vi "Programa_robot_final_2_condicionMala.vi"() -> ()   [LabVIEW 2019]
uses:
  <vilib>/Instr/_visa.llb/VISA Configure Serial Port (Instr).vi
  Global_STOP.vi
  <vilib>/regexp/Match Regular Expression.xnode
panel:
  out "error out":errorcluster
  in  "STOP TEST 2":bool
  out "Datos_QR 2":string
  out "NUMERO ASICS TESTEADOS":i32
  out "Existe foto anterior?":bool
  out ".not. x?":bool
  in  "Config File":path=path "C:/Trabajo/Test Asic Javi_2021/Origen Socket SERVO_PCB_BUENO_v5 (muchos asics)/CONFIG/configuracion_robot_CTAV2022A.test"
  in  "SELECCION DE TEST":string(combo)
  in  "?":bool
  out "Boolean":bool
  in  "Cerrar socket":bool
  in  "Abrir socket":bool
  out "Error_QR":bool
  in  "Interruptor Error":bool
  in  "stop socket 2":bool
  out "Bytes at port 3":u32=1
  in  "IN y":string(combo)="08"
  in  "IN x":string(combo)="06"
  in  "NOK y":string(combo)="00"
  in  "NOK x":string(combo)="00"
  in  "OK y":string(combo)="00"
  in  "OK x":string(combo)="00"
  in  "Operator's name":string(combo)="Juan Rodríguez"
  in  "?":bool
  in  "Fichero de registro":path=path "C:/Trabajo/Pruebas/Pruebas.txt"
  in  "Path Out Report":path=path "C:/Trabajo"
  out "Datos_QR":string
  in  "stop socket":bool
  out "Bytes at port 1":u32
  out "Iteraciones":i32
  out "Lectura buffer":string="1"
  in  "Delay (ms)":dbl=1.0 min=1.0 max=9.0 step=1.0
  out "Bytes at port 2":u32=1
  out "message":string=" INSTRUCTIONS:\r\rNormal Use:  When using subVIs that incorporate the error in/error out (or error I/O) structure, place this handler where you want to inform the user of an error, typically at the end of the I/O data path, as the last action of the program.  If the error in error? is ERROR, the handler creates a message describing the error and its source.  If the type of dialog = 1 (default), the message is displayed to the user, who can only acknowedge it.  If the type = 2, the user can acknowledge the message or abort execution; aborting a program with active I/O is not recommended.  If the type = 0, no message is displayed; this is used to process the error programmatically, and the error out cluster elements are wired to individual terminals for that reason.  \r\rOther Use:\n\r\nlocal testing.  To test the error code of a subVI or function that does not have the error I/O structure, you can wire its error code and a source string to the local error code and error source inputs.  If error in error? indicates no error and error code is not equal to 0, the local code and source are substituted for the error in values, and error? is set TRUE (ERROR)."
  in  "Interruptor":bool=TRUE
  in  "stop":bool
  # "Funcionamiento: en la primera iteración, el efector se desplaza desde el origen hasta la celda\nintroducida, hace una pausa, va a la posición del socket (0,0), hace otra pausa, va a la celda\nde salida y vuelve al origen. En las iteraciones siguientes hará lo mismo pero recorriendo las\nceldas de la bandeja sucesivamente. Que el desplazamiento se produzca hacia una celda de\nla bandeja OK o de la bandeja NOK depende de la salidad del programa de test de Asics."
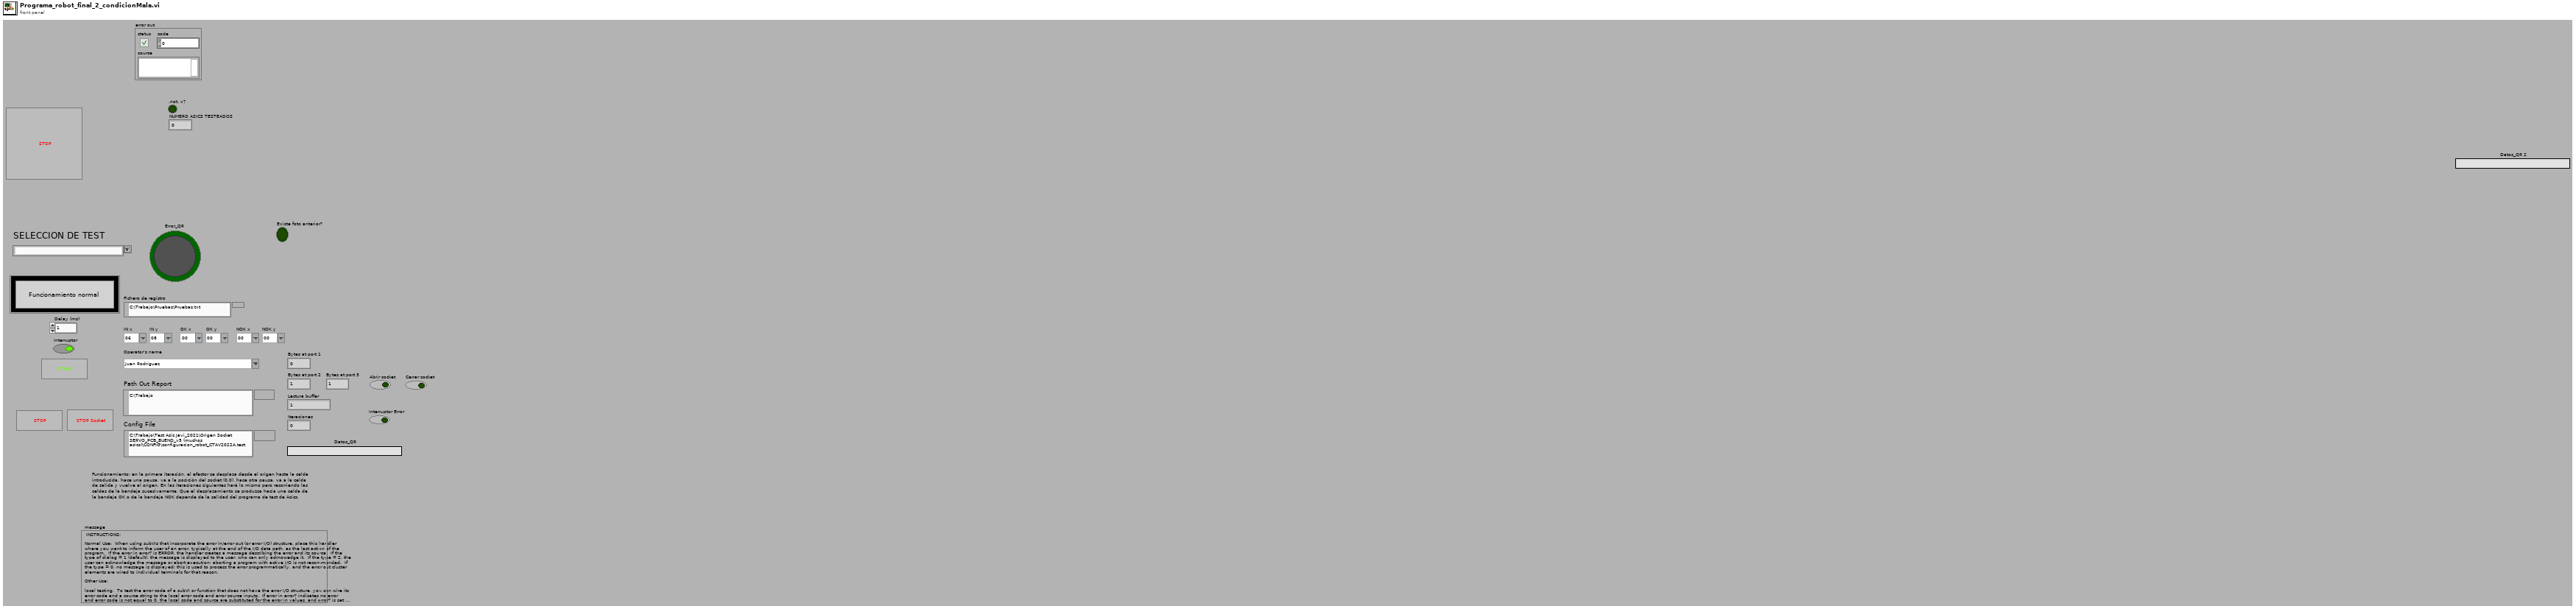
[diagram p1: front panel]
types:
  T1 = enum16{"open", "replace", "create", "open or create", "replace or create", "replace or create with confirmation"}
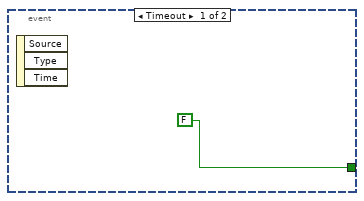
[diagram p2: hidden frame]
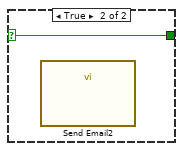
[diagram p3: hidden frame]
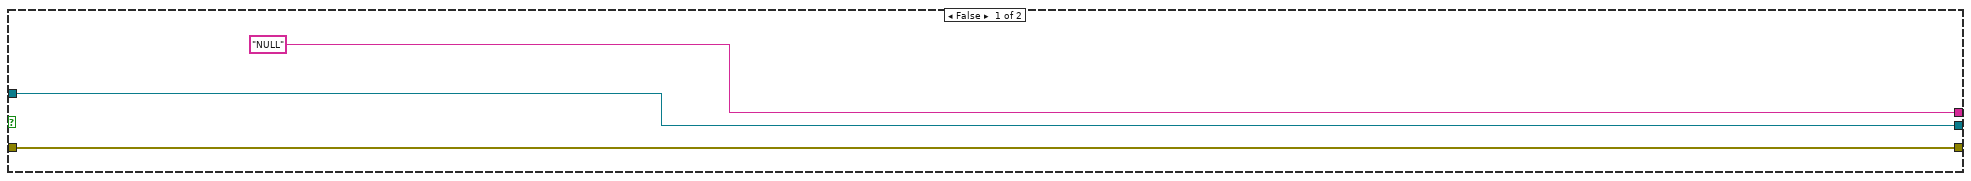
[diagram p4: hidden frame]
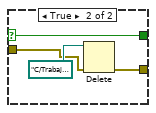
[diagram p7: hidden frame]
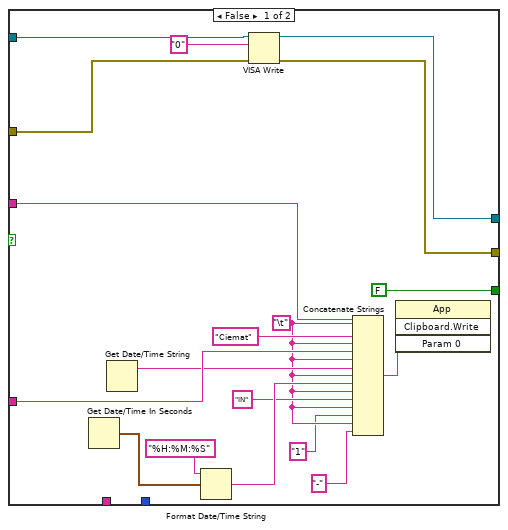
[diagram p9: hidden frame]
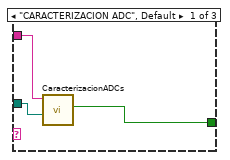
[diagram p10: hidden frame]
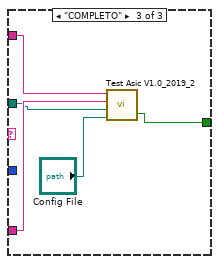
[diagram p11: hidden frame]
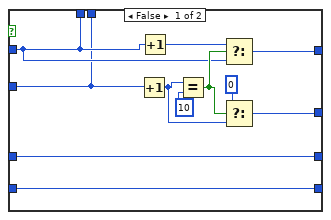
[diagram p13: hidden frame]
diagram:
  # "En el bucle de \"Enviar\" hay que cambiar a modo Latch y quitar la\nnegación para volver al funcionamiento original en el que se avanza\nuna iteración al presionar el botón."
  n1 = flat-sequence {
    tunnel: [w43] -> w5
    tunnel: ["Fichero de registro"] -> w4
    tunnel: ["SELECCION DE TEST"] -> w3
    tunnel: ["NOK y"] -> w20
    tunnel: ["NOK x"] -> w19
    tunnel: ["OK y"] -> w18
    tunnel: ["OK x"] -> w17
    tunnel: ["IN y"] -> w16
    tunnel: ["IN x"] -> w15
    tunnel: [w46] -> w14
    tunnel: [w47] -> w13
    tunnel: ["IN y"] -> w12
    tunnel: ["IN x"] -> w11
    tunnel: w4 -> [w45]
    frame #0 {
      n2 = while {
        stop <- w37 stop-if-true
        n3 = global read "Global_STOP.vi" "stop"() -> (w39:bool)
        n4 = Not(x="?") -> (.not. x?=w40:bool)
        "Boolean" <- w40
        n5 = property on="Boolean" class="Bool (strict)"("Blinking"=w40) -> ()  [unwired: 2 in, 2 out]
        n6 = Or(x="?", y=w39) -> (x .or. y?=w37:bool)
      }
    }
    frame #1 {
      n7 = Not(x="?") -> (.not. x?=w43:bool)
      ".not. x?" <- w43
    }
    frame #2 {
      n8 = Open/Create/Replace File(file path (use dialog)=w45, operation (0:open)=T1."open", access (0:read/write)=enum16{"read/write", "read-only", "write-only"}."write-only") -> (refnum out=w58:refnum<file>, error out=w60:errorcluster)  [unwired: 3 in, 1 out]
      n9 = Set File Position(refnum=w58, from (0:start)=enum16{"start", "end", "current"}."end", error in=w60) -> (refnum out=w59:refnum<file>, error out=w61:errorcluster)  [unwired: 1 in]
      n10 = Write to Text File(file (use dialog)=w59, text="\r\n", error in=w61) -> (refnum out=w47:refnum<file>, error out=w46:errorcluster)  [unwired: 1 in, 1 out]
    }
  }
  n11 = Decimal String To Number(string=w12) -> (number=w10:i32)  [unwired: 2 in, 1 out]
  n12 = Decimal String To Number(string=w11) -> (number=w7:i32)  [unwired: 2 in, 1 out]
  n13 = Multiply(x=10, y=w10) -> (x*y=w8:i32)
  n14 = Decimal String To Number(string=w18) -> (number=w22:i32)  [unwired: 2 in, 1 out]
  n15 = Decimal String To Number(string=w17) -> (number=w21:i32)  [unwired: 2 in, 1 out]
  n16 = Decimal String To Number(string=w20) -> (number=w24:i32)  [unwired: 2 in, 1 out]
  n17 = Decimal String To Number(string=w19) -> (number=w23:i32)  [unwired: 2 in, 1 out]
  n18 = call-poly "VISA Configure Serial Port"("VISA resource name"=refnum<visa-resource-name> "COM4", "baud rate (9600)"=u32 9600, "data bits (8)"=u16 8) -> ("VISA resource name out"=w28:refnum<visa-resource-name>, "error out"=w31:errorcluster)  [unwired: 11 in]
  n19 = Add(x=w8, y=w7) -> (x+y=w6:i32)
  n20 = while {
    shift-right: [w70] -> w29
    shift-left: w31 -> [w112]
    tunnel: w28 -> [w110]
    tunnel: [w73] -> w30
    tunnel: w13 -> [w103]
    tunnel: [w102] -> w27
    tunnel: w14 -> [w101]
    tunnel: [w100] -> w26
    tunnel: w15 -> [w98]
    tunnel: w16 -> [w97]
    tunnel: w17 -> [w96]
    tunnel: w18 -> [w95]
    tunnel: w19 -> [w94]
    tunnel: w20 -> [w93]
    shift-right: [w86] -> _
    shift-left: w24 -> [w92]
    shift-right: [w88] -> _
    shift-left: w23 -> [w91]
    shift-right: [w85] -> _
    shift-left: w22 -> [w90]
    shift-right: [w87] -> _
    shift-left: w21 -> [w89]
    tunnel: w6 -> [w84]
    tunnel: w5 -> [w76]
    tunnel: w3 -> [w75]
    tunnel: [w68] -> w1
    i -> [w74]
    stop <- w68 stop-if-true
    # "Poner Sonda en glbal stop"
    n21 = flat-sequence {
      tunnel: w112 -> [w155]
      tunnel: w110 -> [w144]
      tunnel: [w146] -> w109
      tunnel: [w145] -> w108
      tunnel: w98 -> [w125]
      tunnel: w97 -> [w124]
      tunnel: w96 -> [w123]
      tunnel: w95 -> [w122]
      tunnel: w94 -> [w121]
      tunnel: w93 -> [w120]
      tunnel: w109 -> [w898]
      tunnel: w108 -> [w897]
      tunnel: [w896] -> w83
      tunnel: [w895] -> w81
      tunnel: [w894] -> _
      tunnel: w83 -> [w916]
      tunnel: [w914] -> w82
      tunnel: w81 -> [w915]
      tunnel: [w913] -> w80
      tunnel: w82 -> [w936]
      tunnel: w80 -> [w935]
      tunnel: w74 -> [w937]
      tunnel: [w933] -> w79
      tunnel: [w932] -> w78
      tunnel: [w931] -> w77
      tunnel: w74 -> [w1058]
      tunnel: [w1060] -> w106
      tunnel: [w1059] -> w105
      tunnel: [w1056] -> w99
      tunnel: w79 -> [w1055]
      tunnel: w78 -> [w1054]
      tunnel: w77 -> [w1053]
      tunnel: w76 -> [w1050]
      tunnel: w75 -> [w1048]
      tunnel: w74 -> [w1047]
      tunnel: [w1120] -> w104
      tunnel: [w1122] -> w107
      tunnel: w106 -> [w1121]
      tunnel: w105 -> [w1119]
      tunnel: w103 -> [w1126]
      tunnel: [w1125] -> w102
      tunnel: w101 -> [w1124]
      tunnel: [w1123] -> w100
      tunnel: w74 -> [w1116]
      tunnel: w99 -> [w1115]
      tunnel: w92 -> [w1111]
      tunnel: w91 -> [w1114]
      tunnel: w90 -> [w1113]
      tunnel: w89 -> [w1112]
      tunnel: [w1110] -> w86
      tunnel: [w1109] -> w88
      tunnel: [w1108] -> w85
      tunnel: [w1107] -> w87
      tunnel: w84 -> [w1106]
      tunnel: w74 -> [w1105]
      tunnel: [w1104] -> _
      frame #0 {
        n22 = for {
          N: 2 -> [_]
          shift-right: [w773] -> _
          shift-left: w125 -> [w778]
          shift-right: [w776] -> w141
          shift-left: w144 -> [w777]
          shift-right: [w774] -> w140
          shift-left: w155 -> [w775]
          stop <- w771 stop-if-true
          n23 = xnode "Match Regular Expression"("input string"=w778, "regular expression"="-?\\d") -> ("whole match"=w772:string, "after match"=w773:string)  [unwired: 4 in, 3 out]
          n24 = global read "Global_STOP.vi" "stop"() -> (w771:bool)
          n25 = VISA Write(VISA resource name=w777, write buffer=w772, error in (no error)=w775) -> (VISA resource name out=w776:refnum<visa-resource-name>, error out=w774:errorcluster)  [unwired: 1 out]
        }
        n26 = for {
          N: 2 -> [_]
          shift-right: [w650] -> _
          shift-left: w124 -> [w655]
          shift-right: [w653] -> w135
          shift-left: w141 -> [w654]
          shift-right: [w651] -> w134
          shift-left: w140 -> [w652]
          stop <- w648 stop-if-true
          n27 = xnode "Match Regular Expression"("input string"=w655, "regular expression"="-?\\d") -> ("whole match"=w649:string, "after match"=w650:string)  [unwired: 4 in, 3 out]
          n28 = global read "Global_STOP.vi" "stop"() -> (w648:bool)
          n29 = VISA Write(VISA resource name=w654, write buffer=w649, error in (no error)=w652) -> (VISA resource name out=w653:refnum<visa-resource-name>, error out=w651:errorcluster)  [unwired: 1 out]
        }
        n30 = for {
          N: 2 -> [_]
          shift-right: [w527] -> _
          shift-left: w123 -> [w532]
          shift-right: [w530] -> w137
          shift-left: w135 -> [w531]
          shift-right: [w528] -> w136
          shift-left: w134 -> [w529]
          stop <- w525 stop-if-true
          n31 = xnode "Match Regular Expression"("input string"=w532, "regular expression"="-?\\d") -> ("whole match"=w526:string, "after match"=w527:string)  [unwired: 4 in, 3 out]
          n32 = global read "Global_STOP.vi" "stop"() -> (w525:bool)
          n33 = VISA Write(VISA resource name=w531, write buffer=w526, error in (no error)=w529) -> (VISA resource name out=w530:refnum<visa-resource-name>, error out=w528:errorcluster)  [unwired: 1 out]
        }
        n34 = for {
          N: 2 -> [_]
          shift-right: [w404] -> _
          shift-left: w122 -> [w409]
          shift-right: [w407] -> w129
          shift-left: w137 -> [w408]
          shift-right: [w405] -> w128
          shift-left: w136 -> [w406]
          stop <- w402 stop-if-true
          n35 = xnode "Match Regular Expression"("input string"=w409, "regular expression"="-?\\d") -> ("whole match"=w403:string, "after match"=w404:string)  [unwired: 4 in, 3 out]
          n36 = global read "Global_STOP.vi" "stop"() -> (w402:bool)
          n37 = VISA Write(VISA resource name=w408, write buffer=w403, error in (no error)=w406) -> (VISA resource name out=w407:refnum<visa-resource-name>, error out=w405:errorcluster)  [unwired: 1 out]
        }
        n38 = for {
          N: 2 -> [_]
          shift-right: [w281] -> _
          shift-left: w121 -> [w286]
          shift-right: [w284] -> w131
          shift-left: w129 -> [w285]
          shift-right: [w282] -> w130
          shift-left: w128 -> [w283]
          stop <- w279 stop-if-true
          n39 = xnode "Match Regular Expression"("input string"=w286, "regular expression"="-?\\d") -> ("whole match"=w280:string, "after match"=w281:string)  [unwired: 4 in, 3 out]
          n40 = global read "Global_STOP.vi" "stop"() -> (w279:bool)
          n41 = VISA Write(VISA resource name=w285, write buffer=w280, error in (no error)=w283) -> (VISA resource name out=w284:refnum<visa-resource-name>, error out=w282:errorcluster)  [unwired: 1 out]
        }
        n42 = for {
          N: 2 -> [_]
          shift-right: [w158] -> _
          shift-left: w120 -> [w163]
          shift-right: [w161] -> w127
          shift-left: w131 -> [w162]
          shift-right: [w159] -> w126
          shift-left: w130 -> [w160]
          stop <- w156 stop-if-true
          n43 = xnode "Match Regular Expression"("input string"=w163, "regular expression"="-?\\d") -> ("whole match"=w157:string, "after match"=w158:string)  [unwired: 4 in, 3 out]
          n44 = global read "Global_STOP.vi" "stop"() -> (w156:bool)
          n45 = VISA Write(VISA resource name=w162, write buffer=w157, error in (no error)=w160) -> (VISA resource name out=w161:refnum<visa-resource-name>, error out=w159:errorcluster)  [unwired: 1 out]
        }
        n46 = Number To Decimal String(number="Delay (ms)") -> (decimal integer string=w149:string)  [unwired: 1 in]
        n47 = VISA Write(VISA resource name=w127, write buffer=w149, error in (no error)=w126) -> (VISA resource name out=w151:refnum<visa-resource-name>, error out=w150:errorcluster)  [unwired: 1 out]
        n48 = Select(t="1" ("write buffer"), s="Interruptor", f="0" ("write buffer")) -> (s? t:f=w147:string)
        n49 = VISA Write(VISA resource name=w151, write buffer=w147, error in (no error)=w150) -> (VISA resource name out=w146:refnum<visa-resource-name>, error out=w145:errorcluster)  [unwired: 1 out]
      }
      frame #1 {
        n50 = while {
          shift-right: [w906] -> w895
          shift-left: w897 -> [w911]
          tunnel: ["stop socket"] -> _
          shift-right: [w907] -> w896
          shift-left: w898 -> [w912]
          tunnel: ["stop socket"] -> w894
          stop <- w899 stop-if-true
          n51 = property class="Instr"(reference=w912, error in=w911) -> (reference out=w910:refnum<visa-resource-name>, error out=w909:errorcluster, "Bytes at Port"=w908:u32)
          "Bytes at port 1" <- w908
          n52 = VISA Read(VISA resource name=w910, byte count=w908, error in (no error)=w909) -> (VISA resource name out=w907:refnum<visa-resource-name>, read buffer=w905:string, error out=w906:errorcluster)  [unwired: 1 out]
          n53 = Equal?(x="2", y=w905) -> (x = y?=w903:bool)
          n54 = global read "Global_STOP.vi" "stop"() -> (w900:bool)
          n55 = Or(x=w903, y="stop socket") -> (x .or. y?=w901:bool)
          n56 = Compound Arithmetic op=OR(w901, w900) -> (w899:bool)
        }
      }
      frame #2 {
        n57 = while {
          shift-right: [w924] -> w913
          shift-left: w915 -> [w929]
          tunnel: ["stop socket 2"] -> _
          shift-right: [w925] -> w914
          shift-left: w916 -> [w930]
          tunnel: ["stop socket 2"] -> _
          stop <- w917 stop-if-true
          n58 = property class="Instr"(reference=w930, error in=w929) -> (reference out=w928:refnum<visa-resource-name>, error out=w927:errorcluster, "Bytes at Port"=w926:u32)
          "Bytes at port 3" <- w926
          n59 = VISA Read(VISA resource name=w928, byte count=w926, error in (no error)=w927) -> (VISA resource name out=w925:refnum<visa-resource-name>, read buffer=w923:string, error out=w924:errorcluster)  [unwired: 1 out]
          n60 = Equal?(x="3", y=w923) -> (x = y?=w921:bool)
          n61 = global read "Global_STOP.vi" "stop"() -> (w918:bool)
          n62 = Or(x=w921, y="stop socket 2") -> (x .or. y?=w919:bool)
          n63 = Compound Arithmetic op=OR(w919, w918) -> (w917:bool)
        }
      }
      frame #3 {
        # "Captura y lectura de QR"
        n64 = Greater?(x=w937, y=-1) -> (0:w934:bool)
        n65 = case shown="True" w934 {
          tunnel: [w941 w944] -> w931
          tunnel: w936 -> [w941 w945]
          tunnel: [w940 w943] -> w933
          tunnel: w935 -> [w940 w942]
          tunnel: ["NULL" ("Datos_QR") w946] -> w932
          frame False {
          }
          frame True {
            n66 = while {
              tunnel: [w965] -> w946
              tunnel: w945 -> [w964]
              tunnel: [w960] -> w944
              tunnel: [w959] -> w943
              tunnel: w942 -> [w955]
              stop <- w949 stop-if-true
              n67 = flat-sequence {
                tunnel: w955 -> [w967]
                tunnel: [w968] -> w954
                tunnel: [w981] -> w965
                tunnel: [w979] -> w956
                tunnel: [w978] -> w953
                tunnel: w954 -> [w978]
                frame #0 {
                  n68 = call <vilib>:"Check if File or Folder Exists.vi"("error in (no error)"=w967, "path"=path "C:/Trabajo/Test Asic Javi_2021/Origen Socket SERVO_PCB_BUENO_v5 (muchos asics)/capturaQR.jpg" ("path (use dialog)")) -> ("error out"=w966:errorcluster, "file or folder exists?"=w970:bool, "dup path"=w969:path)  [unwired: 7 in]
                  "Existe foto anterior?" <- w970
                  n69 = case shown="True" w970 {
                    tunnel: w969 -> [w973 w977]
                    tunnel: [w973 w976] -> _
                    tunnel: [w972 w975] -> w968
                    tunnel: w966 -> [w972 w974]
                    frame False {
                    }
                    frame True {
                      n70 = Delete(path (use dialog)=w977, error in=w974) -> (deleted path=w976:path, error out=w975:errorcluster)  [unwired: 3 in, 1 out]
                    }
                  }
                }
                frame #1 {
                  n71 = for {
                    N: 1 -> [_]
                    tunnel: [w986] -> w981
                    tunnel: [w984] -> w979
                    stop <- w982 stop-if-true
                    n72 = call "CapturaImagenyQR_subVI.vi"() -> ("Datos_QR"=w986:string)  [unwired: 11 in]
                    "Datos_QR" <- w986
                    n73 = Equal?(x=w986, y="" ("Datos_QR")) -> (x = y?=w985:bool)
                    n74 = global read "Global_STOP.vi" "stop"() -> (w983:bool)
                    n75 = Not(x=w985) -> (.not. x?=w984:bool)
                    n76 = Compound Arithmetic op=OR(w984, w983) -> (w982:bool)
                  }
                }
              }
              n77 = case shown="False" w956 {
                selector: w956 -> [w989 w993]
                tunnel: [w989 w993] -> w951
                tunnel: w953 -> [w988 w991]
                tunnel: [w988 w990] -> w952
                frame False {
                }
                frame True {
                  n78 = Delete(path (use dialog)=path "C:/Trabajo/Test Asic Javi_2021/Origen Socket SERVO_PCB_BUENO_v5 (muchos asics)/capturaQR.jpg", error in=w991) -> (error out=w990:errorcluster)  [unwired: 3 in, 2 out]
                }
              }
              n79 = Select(t="1" ("write buffer"), s=w951, f="0" ("write buffer")) -> (s? t:f=w961:string)
              n80 = Not(x=w951) -> (.not. x?=w950:bool)
              "Error_QR" <- w950
              n81 = VISA Write(VISA resource name=w964, write buffer=w961, error in (no error)=w952) -> (VISA resource name out=w958:refnum<visa-resource-name>, error out=w957:errorcluster)  [unwired: 1 out]
              n82 = case shown="False" w951 {
                tunnel: w958 -> [w1005 w1046]
                tunnel: w957 -> [w1004 w1045]
                tunnel: [w1003 w1046] -> w960
                tunnel: [w1002 w1045] -> w959
                frame False {
                  n83 = flat-sequence {
                    tunnel: w1005 -> [w1009]
                    tunnel: [w1008] -> w1001
                    tunnel: [w1007] -> w1000
                    tunnel: w1004 -> [w1006]
                    tunnel: w1001 -> [w1022]
                    tunnel: [w1022] -> w999
                    tunnel: w1000 -> [w1021]
                    tunnel: [w1021] -> w998
                    tunnel: w999 -> [w1026]
                    tunnel: w998 -> [w1025]
                    tunnel: [w1024] -> w997
                    tunnel: [w1023] -> w996
                    tunnel: w997 -> [w1039]
                    tunnel: [w1039] -> w995
                    tunnel: w996 -> [w1038]
                    tunnel: [w1038] -> w994
                    tunnel: [w1040] -> w1002
                    tunnel: [w1041] -> w1003
                    tunnel: w995 -> [w1041]
                    tunnel: w994 -> [w1040]
                    frame #0 {
                      n84 = while {
                        tunnel: w1009 -> [w1019]
                        tunnel: [w1015] -> w1008
                        tunnel: [w1014] -> w1007
                        tunnel: w1006 -> [w1013]
                        stop <- w1010 stop-if-true
                        n85 = global read "Global_STOP.vi" "stop"() -> (w1011:bool)
                        n86 = Select(t="2" ("write buffer"), s="Abrir socket", f="0" ("write buffer")) -> (s? t:f=w1016:string)
                        n87 = Or(x="Abrir socket", y=w1011) -> (x .or. y?=w1010:bool)
                        n88 = VISA Write(VISA resource name=w1019, write buffer=w1016, error in (no error)=w1013) -> (VISA resource name out=w1015:refnum<visa-resource-name>, error out=w1014:errorcluster)  [unwired: 1 out]
                      }
                    }
                    frame #1 {
                      n89 = Wait (ms)(milliseconds to wait=u32 1000) -> ()  [unwired: 1 out]
                    }
                    frame #2 {
                      n90 = while {
                        tunnel: w1026 -> [w1033]
                        tunnel: w1025 -> [w1032]
                        tunnel: [w1031] -> w1024
                        tunnel: [w1030] -> w1023
                        stop <- w1027 stop-if-true
                        n91 = global read "Global_STOP.vi" "stop"() -> (w1029:bool)
                        n92 = Select(t="3" ("write buffer"), s="Cerrar socket", f="0" ("write buffer")) -> (s? t:f=w1034:string)
                        n93 = Or(x=w1029, y="Cerrar socket") -> (x .or. y?=w1027:bool)
                        n94 = VISA Write(VISA resource name=w1033, write buffer=w1034, error in (no error)=w1032) -> (VISA resource name out=w1031:refnum<visa-resource-name>, error out=w1030:errorcluster)  [unwired: 1 out]
                      }
                    }
                    frame #3 {
                      n95 = Wait (ms)(milliseconds to wait=u32 1000) -> ()  [unwired: 1 out]
                    }
                    frame #4 {
                      n96 = while {
                        stop <- w1042 stop-if-true
                        n97 = global read "Global_STOP.vi" "stop"() -> (w1043:bool)
                        n98 = Or(x="Interruptor Error", y=w1043) -> (x .or. y?=w1042:bool)
                      }
                    }
                  }
                }
                frame True {
                }
              }
              n99 = global read "Global_STOP.vi" "stop"() -> (w948:bool)
              n100 = Compound Arithmetic op=OR(w951, w948) -> (w949:bool)
              n101 = case shown="True" w950 {
                frame False {
                }
                frame True {
                  n102 = call "Send Email"() -> ()  [unwired: 11 in, 1 out]
                }
              }
            }
            n103 = Wait (ms)(milliseconds to wait=u32 10000) -> ()  [unwired: 1 out]
          }
        }
      }
      frame #4 {
        n104 = Greater?(x=w1058, y=-1) -> (0:w1052:bool)
        n105 = And(x=w1050, y=w1052) -> (x .and. y?=w1051:bool)
        n106 = case shown="True" w1051 {
          tunnel: w1053 -> [w1076 w1088]
          tunnel: w1055 -> [w1075 w1087]
          tunnel: [w1074 w1086] -> w1060
          tunnel: [w1073 w1085] -> w1059
          tunnel: w1054 -> [w1069 w1084]
          tunnel: [FALSE ("Boolean") w1082] -> w1056
          tunnel: "Operator's name" -> [w1067 w1081]
          tunnel: w1048 -> [_ w1080]
          tunnel: w1047 -> [_ w1079]
          frame False {
            w1063 = "\t"
            n107 = Get Date/Time In Seconds() -> (seconds since 1Jan1904=w1071:timestamp)
            n108 = Get Date/Time String() -> (date string=w1066:string)  [unwired: 3 in, 1 out]
            n109 = Format Date/Time String(time format string (%c)="%H:%M:%S", seconds (now)=w1071) -> (date/time string=w1065:string)  [unwired: 1 in]
            n110 = VISA Write(VISA resource name=w1076, write buffer="0", error in (no error)=w1075) -> (VISA resource name out=w1074:refnum<visa-resource-name>, error out=w1073:errorcluster)  [unwired: 1 out]
            n111 = Concatenate Strings(w1069, w1063, "Ciemat", w1063, w1067, w1063, w1066, w1063, w1065, w1063, "IN", w1063, "1", w1063, "-") -> (w1072:string)
            n112 = invoke class="App" method="Clipboard.Write"("Param 0"=w1072) -> ()  [unwired: 3 in, 4 out]
          }
          frame True {
            # "Test de Asics"
            n113 = case shown="\"SUMAS 3 CANALES\"" w1080 {
              tunnel: w1084 -> [w1094 w1096 w1103]
              tunnel: "Path Out Report" -> [w1093 w1098 w1101]
              tunnel: [w1092 w1097 w1099] -> w1082
              tunnel: w1081 -> [_ _ w1102]
              tunnel: w1079 -> [_ w1095 _]
              frame "CARACTERIZACION ADC", Default {
                n114 = call "CaracterizacionADCs.vi"("QR code"=w1094, "Path Out Report"=w1093) -> ("OK/NOK"=w1092:bool)  [unwired: 7 in]
              }
              frame "SUMAS 3 CANALES" {
                n115 = call "Test_Sumadores_Javi.vi"("QR"=w1096, "Path"=w1098, "NUMERO DE PASADA DE TEST"=w1095) -> ("Boolean"=w1097:bool)  [unwired: 8 in]
                "NUMERO ASICS TESTEADOS" <- w1095
              }
              frame "COMPLETO" {
                n116 = call "Test Asic V1.0_2019_2.vi"("Config File"="Config File", "Path Out Report"=w1101, "Operator's Name"=w1102, "ASIC'S Number"=w1103) -> ("OK, Fault 2"=w1099:bool)  [unwired: 1 in]
              }
            }
            n117 = Select(t="1" ("write buffer"), s=w1082, f="0" ("write buffer")) -> (s? t:f=w1089:string)
            n118 = VISA Write(VISA resource name=w1088, write buffer=w1089, error in (no error)=w1087) -> (VISA resource name out=w1086:refnum<visa-resource-name>, error out=w1085:errorcluster)  [unwired: 1 out]
          }
        }
      }
      frame #5 {
        n119 = Greater?(x=w1116, y=-1) -> (0:w1117:bool)
        n120 = case shown="True" w1117 {
          tunnel: w1126 -> [w1132 w1165]
          tunnel: [w1132 w1164] -> w1125
          tunnel: w1124 -> [w1131 w1163]
          tunnel: [w1131 w1162] -> w1123
          tunnel: [w1134 w1161] -> w1122
          tunnel: w1121 -> [w1134 w1161]
          tunnel: [w1133 w1160] -> w1120
          tunnel: w1119 -> [w1133 w1160]
          tunnel: w1115 -> [_ w1158]
          tunnel: w1111 -> [w1130 w1157]
          tunnel: w1114 -> [w1129 w1156]
          tunnel: w1113 -> [w1128 w1155]
          tunnel: w1112 -> [w1127 w1154]
          tunnel: [w1130 w1153] -> w1110
          tunnel: [w1129 w1152] -> w1109
          tunnel: [w1128 w1151] -> w1108
          tunnel: [w1127 w1150] -> w1107
          frame False {
          }
          frame True {
            w1137 = "\t"
            # "Registro de datos en fichero"
            n121 = invoke class="App" method="Clipboard.Read"() -> ("Read Clipbrd"=w1159:string)  [unwired: 3 in, 2 out]
            n122 = case shown="True" w1158 {
              tunnel: w1157 -> [w1168 w1181]
              tunnel: w1156 -> [w1167 w1180]
              tunnel: w1155 -> [w1170 w1178]
              tunnel: w1154 -> [w1169 w1179]
              tunnel: [w1172 w1181] -> w1153
              tunnel: [w1171 w1180] -> w1152
              tunnel: [w1170 w1183] -> w1151
              tunnel: [w1169 w1182] -> w1150
              tunnel: [w1168 w1178] -> w1149
              tunnel: [w1167 w1179] -> w1148
              frame False {
                n123 = Increment(x=w1167) -> (x+1=w1176:i32)
                n124 = Increment(x=w1168) -> (x+1=w1173:i32)
                n125 = Equal?(x=w1176, y=10) -> (x = y?=w1174:bool)
                n126 = Select(t=w1173, s=w1174, f=w1168) -> (s? t:f=w1172:i32)
                n127 = Select(t=0, s=w1174, f=w1176) -> (s? t:f=w1171:i32)
              }
              frame True {
                n128 = Increment(x=w1179) -> (x+1=w1187:i32)
                n129 = Increment(x=w1178) -> (x+1=w1184:i32)
                n130 = Equal?(x=w1187, y=10) -> (x = y?=w1185:bool)
                n131 = Select(t=w1184, s=w1185, f=w1178) -> (s? t:f=w1183:i32)
                n132 = Select(t=0, s=w1185, f=w1187) -> (s? t:f=w1182:i32)
              }
            }
            n133 = Write to Text File(file (use dialog)=w1165, text=w1159, error in=w1163) -> (refnum out=w1146:refnum<file>, error out=w1147:errorcluster)  [unwired: 1 in, 1 out]
            n134 = Number To Decimal String(number=w1149) -> (decimal integer string=w1136:string)  [unwired: 1 in]
            n135 = Number To Decimal String(number=w1148) -> (decimal integer string=w1135:string)  [unwired: 1 in]
            n136 = Write to Text File(file (use dialog)=w1146, text=w1137, error in=w1147) -> (refnum out=w1144:refnum<file>, error out=w1145:errorcluster)  [unwired: 1 in, 1 out]
            n137 = Write to Text File(file (use dialog)=w1144, text=w1136, error in=w1145) -> (refnum out=w1141:refnum<file>, error out=w1140:errorcluster)  [unwired: 1 in, 1 out]
            n138 = Write to Text File(file (use dialog)=w1141, text=w1137, error in=w1140) -> (refnum out=w1139:refnum<file>, error out=w1138:errorcluster)  [unwired: 1 in, 1 out]
            n139 = Write to Text File(file (use dialog)=w1139, text=w1135, error in=w1138) -> (refnum out=w1143:refnum<file>, error out=w1142:errorcluster)  [unwired: 1 in, 1 out]
            n140 = Write to Text File(file (use dialog)=w1143, text="\r\n", error in=w1142) -> (refnum out=w1164:refnum<file>, error out=w1162:errorcluster)  [unwired: 1 in, 1 out]
          }
        }
        n141 = Add(x=w1106, y=w1105) -> (x+y=w1104:i32)
      }
    }
    n142 = while {
      shift-right: [w1196] -> w72
      shift-left: w104 -> [w1202]
      tunnel: ["stop"] -> _
      shift-right: [w1197] -> w73
      shift-left: w107 -> [w1203]
      tunnel: [w1192] -> w111
      stop <- w1190 stop-if-true
      # "1"
      # "Mientras se ejecuta este bucle (la espera a que\nArduino termine una iteración), cambiamos los\ndatos de los controladores."
      n143 = property class="Instr"(reference=w1203, error in=w1202) -> (reference out=w1200:refnum<visa-resource-name>, error out=w1199:errorcluster, "Bytes at Port"=w1198:u32)
      "Bytes at port 2" <- w1198
      n144 = VISA Read(VISA resource name=w1200, byte count=w1198, error in (no error)=w1199) -> (VISA resource name out=w1197:refnum<visa-resource-name>, read buffer=w1192:string, return count=w1195:u32, error out=w1196:errorcluster)
      n145 = Greater Or Equal?(x=w1195, y=u32 1) -> (x >= y?=w1193:bool)
      n146 = global read "Global_STOP.vi" "stop"() -> (w1189:bool)
      n147 = Or(x=w1193, y="stop") -> (x .or. y?=w1191:bool)
      n148 = Compound Arithmetic op=OR(w1191, w1189) -> (w1190:bool)
    }
    "Lectura buffer" <- w111
    n149 = for {
      N: 3 -> [_]
      tunnel: [w118] -> _
      tunnel: [w115] -> w69
      tunnel: w72 -> [w116]
      tunnel: [w116] -> w64
      tunnel: [w115] -> w63
      stop <- w115 stop-if-true
      n150 = call "CapturaImagenyQR_subVI.vi"() -> ("Datos_QR"=w118:string)  [unwired: 11 in]
      "Datos_QR 2" <- w118
      n151 = Equal?(x=w118, y="" ("Datos_QR")) -> (x = y?=w117:bool)
      n152 = Not(x=w117) -> (.not. x?=w115:bool)
    }
    n153 = global read "Global_STOP.vi" "stop"() -> (w62:bool)
    n154 = Or(x=w62, y=w63) -> (x .or. y?=w68:bool)
    n155 = Boolean To (0,1)(Boolean=w69) -> (0, 1=w66:i16)
    n156 = call <vilib>:"Error Cluster From Error Code.vi"("error in (no error)"=w64, "error message (\"\")"="El asic no se ha colocado en la\n  bandeja de salida,se ha quedado\nen el socket posiblemente por una\nmala succión de la ventosa.\nPulsar el boton STOP." ("error message (\"\")"), "error code (0)"=w66) -> ("error out"=w65:errorcluster)  [unwired: 6 in]
    n157 = call <vilib>:"Simple Error Handler.vi"("error in (no error)"=w65) -> ("error out"=w70:errorcluster)  [unwired: 4 in, 4 out]
    n158 = case shown="False" w69 {
      selector: w69 -> [w113 w114]
      tunnel: [w113 w114] -> _
      frame False {
      }
      frame True {
        n159 = call "Send Email2"() -> ()  [unwired: 11 in, 1 out]
      }
    }
    "Iteraciones" <- w74
  }
  n160 = flat-sequence {
    frame #0 {
      n161 = local write "STOP TEST 2"(FALSE ("STOP TEST 2")) -> ()
    }
    frame #1 {
      n162 = while {
        stop <- w1205 stop-if-true
        n163 = event shown="[1] \"STOP TEST 2\": Value Change" {
          selector: _ -> [_ _]
          dyn-events: _ -> [_ _]
          timeout: _ -> [_ _]
          tunnel: [FALSE "STOP TEST 2"] -> w1205
          event Timeout {
            n164 = event-data() -> ()  [unwired: 1 in, 3 out]
          }
          event "STOP TEST 2": Value Change {
            n165 = event-data() -> ()  [unwired: 1 in, 6 out]
            n166 = global write "Global_STOP.vi" "stop"("STOP TEST 2") -> ()
            n167 = Wait (ms)(milliseconds to wait=u32 100) -> ()  [unwired: 1 out]
          }
        }
      }
    }
  }
  n168 = Close File(refnum=w27, error in=w26) -> (error out=w25:errorcluster)  [unwired: 1 out]
  n169 = Not(x=w1) -> (.not. x?=w2:bool)
  n170 = call <vilib>:"Simple Error Handler.vi"("error in (no error)"=w25) -> ()  [unwired: 4 in, 5 out]
  n171 = global write "Global_STOP.vi" "stop"(w2) -> ()
  n172 = VISA Close(VISA resource name=w30, error in (no error)=w29) -> (error out=w35:errorcluster)
  "error out" <- w35
  n173 = call <vilib>:"Simple Error Handler.vi"("error in (no error)"=w35) -> ("message"=→"message":string)  [unwired: 4 in, 4 out]
